vi "Test_HSDIO_AWG_Standalone_Async.vi"(8 "error in (no error)":errorcluster, 10 "AWG 5421 Inputs":T6={"Resource Name"="AWG_5421", "Sample Rate"=10000000.0, "Trigger Type"=2, "Trigger Source"="PFI0"} {"Sample Rate" format="%.2p"; "Trigger Type" items=["None", "Software Edge", "Digital Edge", "Digital Level"]}) -> (0 "error out":errorcluster)   [LabVIEW 2015]
doc: "This VI inits a waveform generation session for AWG-5421. This is a basic example that shows how to setup the board in order to generate waveforms according to a script. \nBy default this configuration uses one channel CH0, and one script trigger ScriptTrigger0. The ScriptTrigger0 is waiting for an external trigger : i.e. a digital Edge on pin PFI 0 by default.\n\nThere are various options for the script to be used. Consult the Script control help for more information on configuring the example for specific scripts."
uses:
  controls/AWG_5421_Inputs.ctl
  <instrlib>/niFgen/niFgen.llb/niFgen_ctl Trigger Source Values (Ring).ctl
  controls/HSDIO_6541_Inputs.ctl
  <instrlib>/niHSDIO/niHSDIO.llb/niHSDIO_ctl Trigger Source Values (Ring).ctl
  controls/TIMING_Inputs.ctl
  controls/SOFTWARE_Inputs.ctl
panel:
  in  "EXCIT Inputs":T1={"Number of Excitations"=1, "Script text"="script myScript0\n    wait until scriptTrigger0\n    Generate Sinus250to250a100dur800fs10\nend script", "Table of Waveforms"=["Sinus250to250a100dur800fs10"]} {"Number of Excitations" min=1 max=10}
  in  "SOFTWARE Inputs":T2={"Application Directory"=path "D:/S.O.F.T.S/LABVIEW/PIL", "Resources Path"=path "D:/S.O.F.T.S/LABVIEW/PIL/resources", "Data Path"=path "D:/PIRENEA/DATA", "XML Path"=path "D:/PIRENEA/DATA", "XML File Filter"="*.xml", "Excit Scripts Path"=path "D:/PIRENEA/EXCIT_SCRIPTS", "Excit Scripts File Filter"="*.txt", "Excit Waveforms Path"=path "D:/PIRENEA/EXCIT_WFMS", "Excit Waveforms File Filter"="*.bin", "Timing Scripts Path"=path "D:/PIRENEA/TIMING_SCRIPTS", "Timing Scripts File Filter"="*.txt", "Timing Waveforms Path"=path "D:/PIRENEA/TIMING_WFMS", "Timing Waveforms File Filter"="*.bin", "Trapping Waveforms Path"=path "D:/PIRENEA/TRAPPING_WFMS", "Trapping Waveforms File Filter"="*.bin"}
  in  "TIMING Inputs":T3={"Number of Acquisitions "=1, "Number of Accumulations"=1, "Table of Waveforms"=[], "Script Text"=""} {"Number of Accumulations" min=0 max=50 step=1; "Number of Acquisitions" min=1 max=10 step=1}
  in  "HSDIO 6541 Inputs":T4={"Resource Name"="HSDIO_6541", "Clock Rate"=1000000.0, "Trigger Source"="PFI0"} {"Clock Rate" format="%.2p"}
  in  "Script 2 (NOT USED)":string="script myScript0\n    wait until scriptTrigger0\n    Generate Sinus250to250a100dur800fs10\nend script"
  # "ATTENTION\nModifier Sample Rate\nen fonction de la forme\nqui est codee en dur dans le\ndiagramme !!!"
  # "ATTENTION\nsi wait until scriptTrigger0 dans le\nscript alors obligatoirement\nattente d'un trigger (soft ou hard)"
  # "ATTENTION\nsi AUCUN wait until scriptTrigger0\ndans le script alors generation\nimmediate de la waveform"
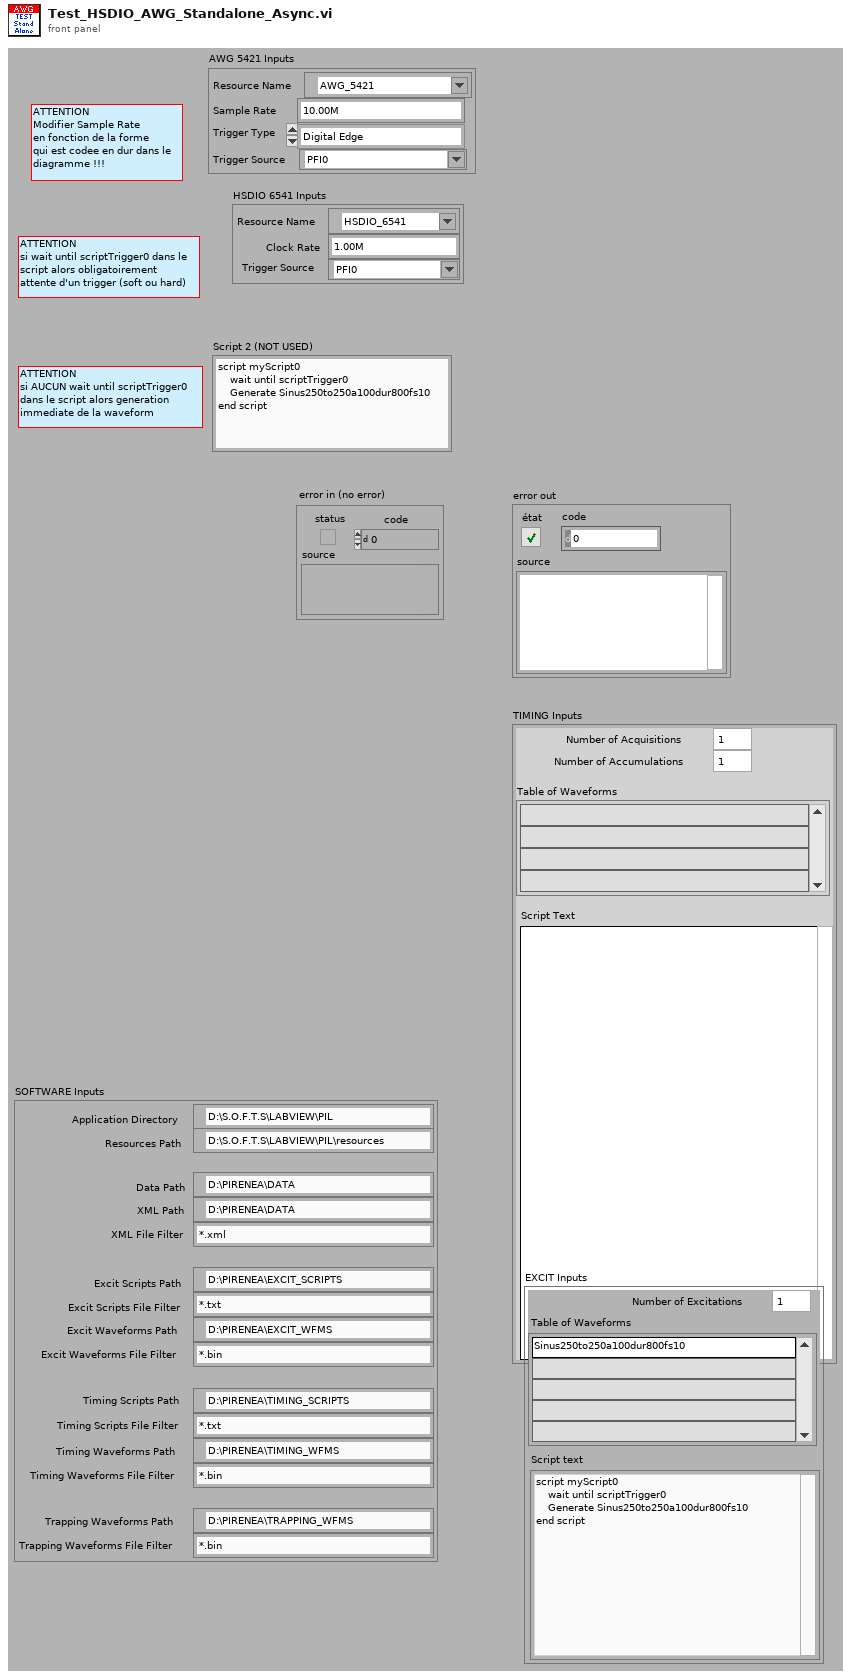
[diagram p1: front panel]
types:
  T1 = cluster{"Number of Excitations":i32, "Script text":string, "Table of Waveforms":string[]}
  T2 = typedef "SOFTWARE_Inputs.ctl" = cluster{"Application Directory":path, "Resources Path":path, "Data Path":path, "XML Path":path, "XML File Filter":string, "Excit Scripts Path":path, "Excit Scripts File Filter":string, "Excit Waveforms Path":path, "Excit Waveforms File Filter":string, "Timing Scripts Path":path, "Timing Scripts File Filter":string, "Timing Waveforms Path":path, "Timing Waveforms File Filter":string, "Trapping Waveforms Path":path, "Trapping Waveforms File Filter":string}
  T3 = typedef "TIMING_Inputs.ctl" = cluster{"Number of Acquisitions ":i16, "Number of Accumulations":i16, "Table of Waveforms":string[], "Script Text":string}
  T4 = typedef "HSDIO_6541_Inputs.ctl" = cluster{"Resource Name":refnum<k15>, "Clock Rate":dbl, "Trigger Source":T5}
  T5 = typedef "niHSDIO_ctl Trigger Source Values (Ring).ctl" = string
  T6 = typedef "AWG_5421_Inputs.ctl" = cluster{"Resource Name":refnum<k15>, "Sample Rate":dbl, "Trigger Type":u16, "Trigger Source":T7}
  T7 = typedef "niFgen_ctl Trigger Source Values (Ring).ctl" = string
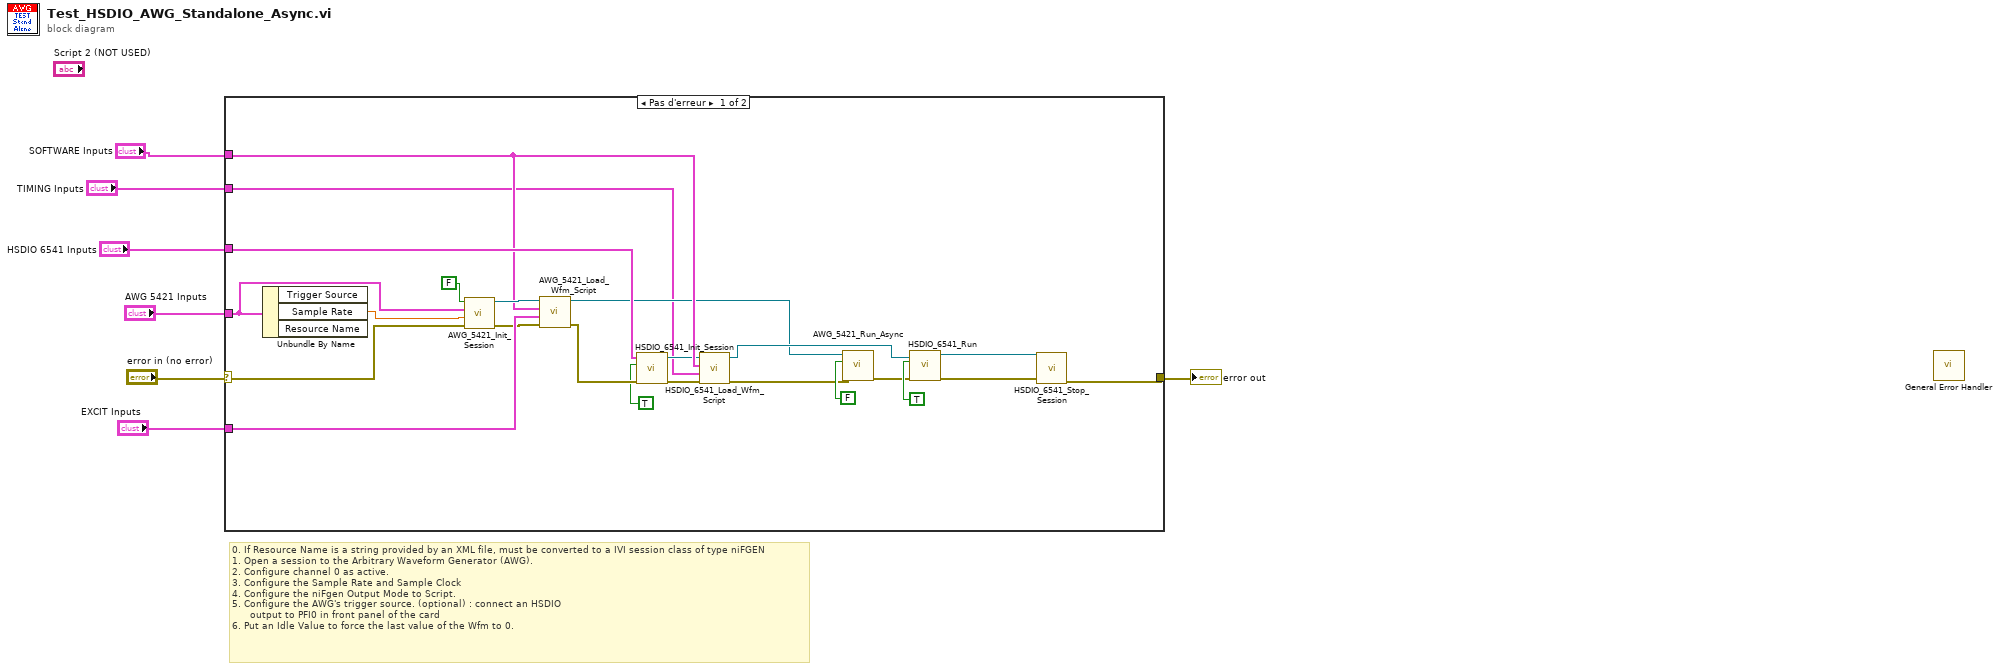
[diagram p0: block diagram]
diagram:
  # "0. If Resource Name is a string provided by an XML file, must be converted to a IVI session class of type niFGEN\n1. Open a session to the Arbitrary Waveform Generator (AWG).\n2. Configure channel 0 as active. \n3. Configure the Sample Rate and Sample Clock\n4. Configure the niFgen Output Mode to Script.\n5. Configure the AWG's trigger source. (optional) : connect an HSDIO\n      output to PFI0 in front panel of the card \n6. Put an Idle Value to force the last value of the Wfm to 0."
  n1 = case shown="Pas d'erreur" "error in (no error)" {
    selector: "error in (no error)" -> [w27 w31]
    tunnel: [w22 w31] -> w7
    tunnel: "AWG 5421 Inputs" -> [w29 _]
    tunnel: "HSDIO 6541 Inputs" -> [w20 _]
    tunnel: "EXCIT Inputs" -> [w26 _]
    tunnel: "SOFTWARE Inputs" -> [w17 _]
    tunnel: "TIMING Inputs" -> [w8 _]
    frame No Error {
      n2 = Unbundle By Name(w29) -> ("Sample Rate"=w28:dbl)  [unwired: 2 out]
      n3 = call "AWG_5421_Init_Session.vi"("error in (no error)"=w27, "Sample Rate"=w28, "AWG 5421 Inputs"=w29, "Use Software Trigger"=FALSE) -> ("error out"=w24:errorcluster, "Instrument handle out"=w25:refnum<k15>)  [unwired: 6 in]
      n4 = call "AWG_5421_Load_Wfm_Script.vi"("error  in"=w24, "EXCIT Inputs"=w26, "SOFTWARE Inputs"=w17, "instrument handle in"=w25) -> ("error out"=w21:errorcluster, "instrument handle out"=w9:refnum<k15>)  [unwired: 3 in, 3 out]
      n5 = call "HSDIO_6541_Init_Session.vi"("error in (no error)"=w21, "Use Software Trigger"=TRUE, "HSDIO 6541 Inputs"=w20) -> ("error out"=w18:errorcluster, "instrument handle out"=w16:refnum<k15>)  [unwired: 7 in]
      n6 = call "HSDIO_6541_Load_Wfm_Script.vi"("error  in"=w18, "TIMING Inputs"=w8, "SOFTWARE Inputs"=w17, "instrument handle in"=w16) -> ("error out"=w15:errorcluster, "instrument handle out"=w14:refnum<k15>)  [unwired: 4 in, 2 out]
      n7 = call "AWG_5421_Run_Async.vi"("error in (no error)"=w15, "Use Software trigger"=FALSE, "AWG5421 Resource Name"=w9) -> ("error out"=w12:errorcluster)  [unwired: 8 in]
      n8 = call "HSDIO_6541_Run.vi"("error  in"=w12, "Use Software trigger"=TRUE, "instrument handle in"=w14) -> ("error out"=w10:errorcluster, "instrument handle out"=w11:refnum<k15>)  [unwired: 7 in]
      n9 = call "HSDIO_6541_Stop_Session.vi"("error in (no error)"=w10, "instrument handle in"=w11) -> ("error out"=w22:errorcluster)  [unwired: 9 in]
    }
    frame Error {
    }
  }
  "error out" <- w7
  n10 = call <vilib>:"General Error Handler.vi"() -> ()  [unwired: 11 in, 5 out]
